vi "DBL Array Test.vi"() -> ()   [LabVIEW 2013]
uses:
  <vilib>/dlg_ctls.llb/Space Constant.vi
  subVIs/JSON No Whitespace.vi
  <vilib>/Utility/error.llb/Trim Whitespace.vi
  LV JSON.lvlib
panel:
  out "variant":variant
  out "data 2":dbl[](array[numeric])
  out "DBLArray":string
  in  "DBLarray":dbl[](array[numeric])=[1.0, 2.0, 3.0]
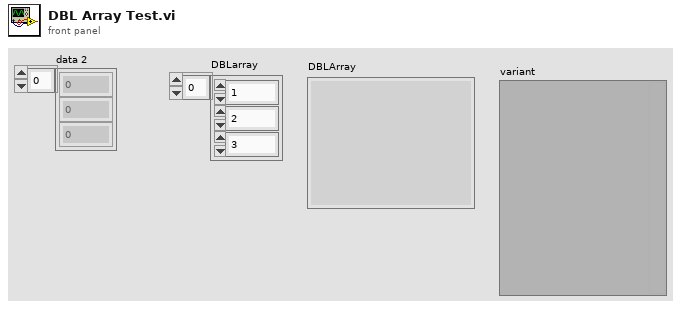
[diagram p1: front panel]
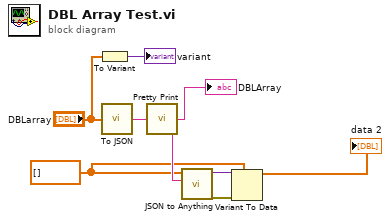
[diagram p0: block diagram]
diagram:
  w1 = dbl[] [] ("DBLarray")
  n1 = To Variant(anything="DBLarray") -> (Variant=→"variant":variant)
  n2 = call "To JSON.vi"("Anything"="DBLarray") -> ("JSON"=w8:string)  [unwired: 1 in]
  n3 = call "Pretty Print.vi"("JSON String"=w8) -> ("Pretty JSON String"=w7:string)  [unwired: 1 out]
  "DBLArray" <- w7
  n4 = call "JSON to Anything.vi"("JSON Object"=w7, "Type"=w1) -> ("error out"=w5:errorcluster, "Variant"=w4:variant)  [unwired: 6 in, 2 out]
  n5 = Variant To Data(error in=w5, type=w1, Variant=w4) -> (data=→"data 2":dbl[])  [unwired: 1 out]
